vi "_AdjustDelayTime.vi"(5 "CombinedModeAndPol":bool, 6 "SourceProperty in":T1[](array[typedef]) {"Source Type" items=["APCI 1", "APCI 2", "ESI 1", "ESI 2"]}, 7 "ExptList":i32[](array[numeric])) -> (2 "SourceProperty out":T1[](array[typedef]) {"Source Type" items=["APCI 1", "APCI 2", "ESI 1", "ESI 2"]})   [LabVIEW 2012]
uses:
  _Source Properties.ctl
  _XML Source Type.ctl
  Configuration/_Global Configuration.vi
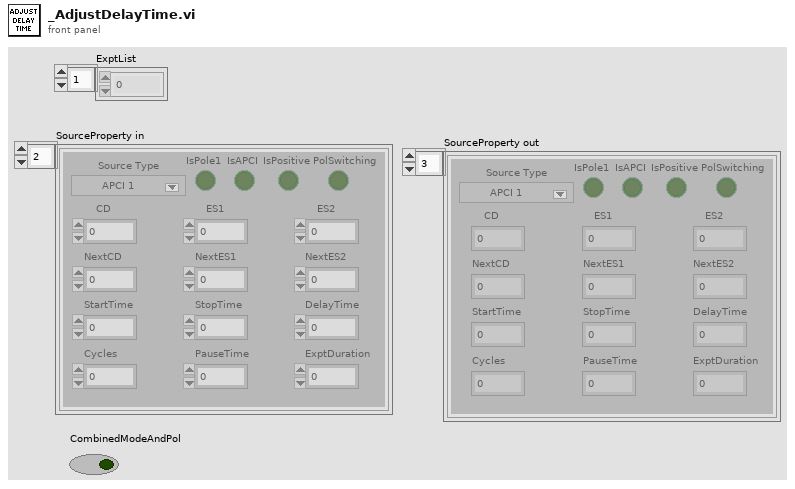
[diagram p1: front panel]
types:
  T1 = typedef "_Source Properties.ctl" = cluster{"Source Type":T2, "IsPole1":bool, "IsAPCI":bool, "IsPositive":bool, "CD":dbl, "ES1":dbl, "ES2":dbl, "NextCD":dbl, "NextES1":dbl, "NextES2":dbl, "PolSwitching":bool, "StartTime":dbl, "StopTime":dbl, "DelayTime":dbl, "Cycles":i32, "PauseTime":dbl, "ExptDuration":dbl}
  T2 = typedef "_XML Source Type.ctl" = u16
  T3 = typedef "_RT Instrument 2.ctl" = cluster{"Table":T4[], "Instrument":string[]}
  T4 = typedef "_RT Configuration 2.ctl" = cluster{"Name":string, "Ch#":u8, "Min":dbl, "Max":dbl, "Def+":dbl, "Def-":dbl, "Offset":dbl, "Slope":dbl, "Type":u8, "Description":string, "SettleT":dbl}
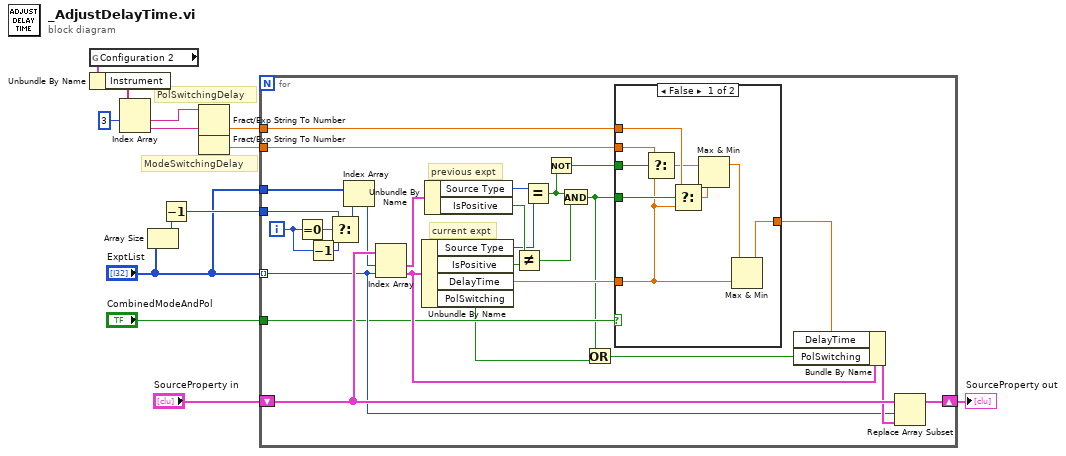
[diagram p0: block diagram]
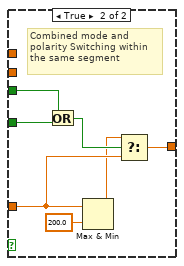
[diagram p2: hidden frame]
diagram:
  # "PolSwitchingDelay"
  # "ModeSwitchingDelay"
  n1 = global read "_Global Configuration.vi" "Configuration 2"() -> (w5:T3)
  n2 = Unbundle By Name(w5) -> ("Instrument"=w6:string[])
  n3 = Index Array(array=w6, index #1=3 ("index")) -> (element #1=w8:string, element #2=w9:string)  [unwired: 1 in]
  n4 = Array Size(array="ExptList") -> (size(s)=w11:i32)
  n5 = Decrement(x=w11) -> (x-1=w2:i32)
  n6 = Fract/Exp String To Number(string=w8) -> (number=w4:dbl)  [unwired: 3 in, 1 out]
  n7 = Fract/Exp String To Number(string=w9) -> (number=w3:dbl)  [unwired: 3 in, 1 out]
  n8 = for {
    shift-right: [w39] -> w13
    shift-left: "SourceProperty in" -> [w41]
    tunnel: "ExptList" -> [w35] mode=indexing
    tunnel: w2 -> [w33]
    tunnel: "CombinedModeAndPol" -> [w22]
    tunnel: w4 -> [w21]
    tunnel: w3 -> [w20]
    tunnel: "ExptList" -> [w15]
    i -> [w34]
    # "current expt"
    # "previous expt"
    n9 = Equal To 0?(x=w34) -> (x = 0?=w37:bool)
    n10 = Decrement(x=w34) -> (x-1=w36:i32)
    n11 = Select(t=w33, s=w37, f=w36) -> (s? t:f=w16:i32)
    n12 = Index Array(array=w15, index=w16) -> (element=w14:i32)
    n13 = Index Array(array=w41, index #1=w14, index #2=w35) -> (element #1=w32:T1, element #2=w24:T1)
    n14 = Unbundle By Name(w24) -> ("Source Type"=w28:T2, "IsPositive"=w31:bool, "DelayTime"=w23:dbl, "PolSwitching"=w17:bool)
    n15 = Unbundle By Name(w32) -> ("Source Type"=w29:T2, "IsPositive"=w30:bool)
    n16 = Not Equal?(x=w30, y=w31) -> (x != y?=w27:bool)
    n17 = Equal?(x=w29, y=w28) -> (x = y?=w25:bool)
    n18 = Not(x=w25) -> (.not. x?=w26:bool)
    n19 = And(x=w25, y=w27) -> (x .and. y?=w19:bool)
    n20 = Or(x=w19, y=w17) -> (x .or. y?=w18:bool)
    n21 = case shown="False" w22 {
      tunnel: [w42 w56] -> w38
      tunnel: w26 -> [w50 w55]
      tunnel: w19 -> [w48 w53]
      tunnel: w23 -> [w43 w52]
      tunnel: w21 -> [w47 _]
      tunnel: w20 -> [w49 _]
      frame False {
        n22 = Select(t=w49, s=w50, f=w43) -> (s? t:f=w46:dbl)
        n23 = Select(t=w47, s=w48, f=w43) -> (s? t:f=w45:dbl)
        n24 = Max & Min(x=w46, y=w45) -> (max(x,y)=w44:dbl)  [unwired: 1 out]
        n25 = Max & Min(x=w44, y=w43) -> (max(x,y)=w42:dbl)  [unwired: 1 out]
      }
      frame True {
        # "Combined mode and\npolarity Switching within\nthe same segment"
        n26 = Or(x=w55, y=w53) -> (x .or. y?=w54:bool)
        n27 = Max & Min(x=w52, y=200.0) -> (max(x,y)=w51:dbl)  [unwired: 1 out]
        n28 = Select(t=w51, s=w54, f=w52) -> (s? t:f=w56:dbl)
      }
    }
    n29 = Bundle By Name(cluster=w24, "DelayTime"=w38, "PolSwitching"=w18) -> (w40:T1)
    n30 = Replace Array Subset(array=w41, new element=w40, index=w35) -> (w39:T1[])
  }
  "SourceProperty out" <- w13
